vi "set_config_cluster.vi"(8 "error in (no error)":errorcluster, 10 "config cluster variant":variant, 11 "LightSourceMH110124MaiTai in":refnum<class "LightSourceMH110124MaiTai.lvclass">) -> (0 "error out":errorcluster, 3 "LightSourceMH110124MaiTai out":refnum<class "LightSourceMH110124MaiTai.lvclass">)   [LabVIEW 2010, in "LightSourceMH110124MaiTai.lvclass"]
uses:
  LightSourceMH110124MaiTai.lvclass
  LightSourceMH110124MaiTai.lvclass/LightSourceMH110124MaiTai.ctl
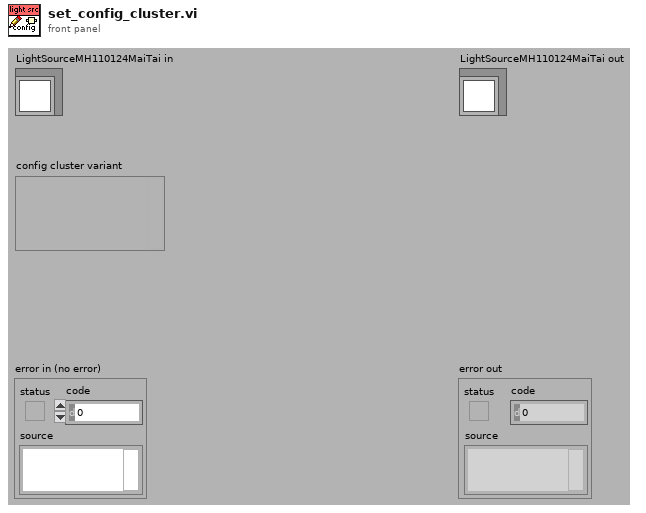
[diagram p1: front panel]
types:
  T1 = typedef "LightSourceMH110124MaiTai.lvclass/config_data_cluster.ctl" = cluster{"hardware settings":cluster{"comm port":string, "switch laser on?":bool, "open shutter?":bool, "wavelength":dbl[unit], "delay before read (ms)":u32, "flow control":u16, "stop bits":u16, "data bits":u16, "baud rate":u32, "parity (0:none)":enum16{"None", "Odd", "Even", "Mark", "Space"}}}
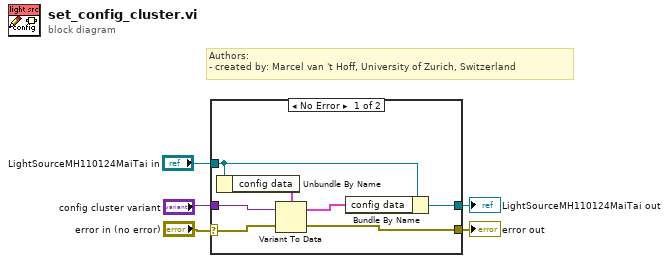
[diagram p0: block diagram]
diagram:
  # "Authors: \n- created by: Marcel van 't Hoff, University of Zurich, Switzerland"
  n1 = case shown="No Error" "error in (no error)" {
    selector: "error in (no error)" -> [w10 w14]
    tunnel: [w6 w14] -> w1
    tunnel: [w7 w13] -> w2
    tunnel: "LightSourceMH110124MaiTai in" -> [w9 w13]
    tunnel: "config cluster variant" -> [w11 _]
    frame No Error {
      n2 = Unbundle By Name(w9) -> ("config data"=w12:T1)
      n3 = Variant To Data(error in=w10, Variant=w11, type=w12) -> (error out=w6:errorcluster, data=w8:T1)
      n4 = Bundle By Name(cluster=w9, "config data"=w8) -> (w7:refnum<class "LightSourceMH110124MaiTai.lvclass">)
    }
    frame Error {
    }
  }
  "error out" <- w1
  "LightSourceMH110124MaiTai out" <- w2
